vi "Get DVR From Circular Buffer.vi"(8 "error in (no error)":errorcluster, 10 "Ignore Read Lock":bool, 11 "CIF_NIChn_Fifo_Power_DVR in":refnum<class "CIF_NIChn_Fifo_Power_DVR.lvclass">) -> (0 "error out":errorcluster, 1 "Timeout":bool, 2 "DVRs":refnum<data-value>[](array[refnum]), 3 "CIF_NIChn_Fifo_Power_DVR out":refnum<class "CIF_NIChn_Fifo_Power_DVR.lvclass">)   [LabVIEW 2021, in "CIF_NIChn_Fifo_Power_DVR.lvclass"]
uses:
  CIF_NIChn_Fifo_Power_DVR.lvclass
  CIF_NIChn_Fifo_Power_DVR.lvclass/CIF_NIChn_Fifo_Power_DVR.ctl
  ChannelCommon/ChannelCommon.lvlib
  ChannelCommon/typedef/Datatype Waveform.ctl
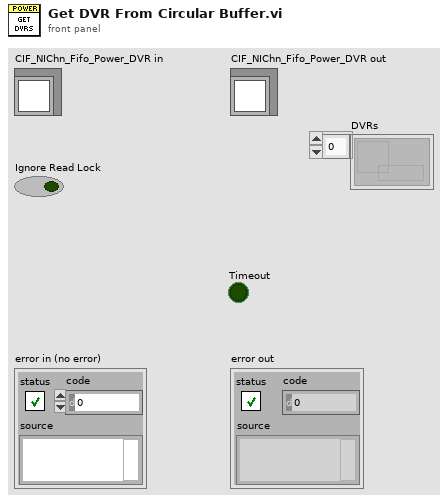
[diagram p1: front panel]
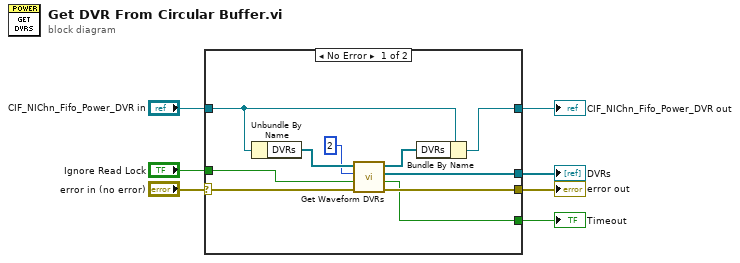
[diagram p0: block diagram]
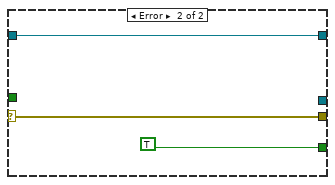
[diagram p2: hidden frame]
diagram:
  n1 = case shown="No Error" "error in (no error)" {
    selector: "error in (no error)" -> [w14 w20]
    tunnel: [w13 w20] -> w6
    tunnel: [w16 w19] -> w4
    tunnel: "CIF_NIChn_Fifo_Power_DVR in" -> [w17 w19]
    tunnel: "Ignore Read Lock" -> [w8 _]
    tunnel: [w11 _] -> w1
    tunnel: [w10 TRUE ("Read Lock")] -> w2
    frame No Error {
      n2 = Unbundle By Name(w17) -> ("DVRs"=w15:refnum<data-value>[])
      n3 = call "Get Waveform DVRs.vi"("error in (no error)"=w14, "Ignore Read Lock"=w8, "Number of Waveforms"=2, "DVR Circular Buffer in"=w15) -> ("error out"=w13:errorcluster, "Timeout"=w10:bool, "DVRs"=w11:refnum<data-value>[], "DVR Circular Buffer out"=w12:refnum<data-value>[])  [unwired: 4 in]
      n4 = Bundle By Name(cluster=w17, "DVRs"=w12) -> (w16:refnum<class "CIF_NIChn_Fifo_Power_DVR.lvclass">)
    }
    frame Error {
    }
  }
  "error out" <- w6
  "CIF_NIChn_Fifo_Power_DVR out" <- w4
  "Timeout" <- w2
  "DVRs" <- w1
